vi "Add_Image_Position_Offset.vi"() -> (5 "Plug in titles":string[](array[string]), 7 "Plug in values":string[](array[string]))   [LabVIEW 2020]
uses:
  Utilities/Image acquisition and processing/Feature detection/Typedefs/Theta range.ctl
  Utilities/Image acquisition and processing/Feature detection/Typedefs/Txy range.ctl
  Globals/Meas_global.vi
  Globals/Extra_Commands_Global.vi
  Globals/Trav_pos_global.vi
panel:
  in  "Pre-scale iters":i32=2
  in  "R_min":dbl=200.0
  out "Ty (pixels)":dbl
  out "Tx (pixels)":dbl
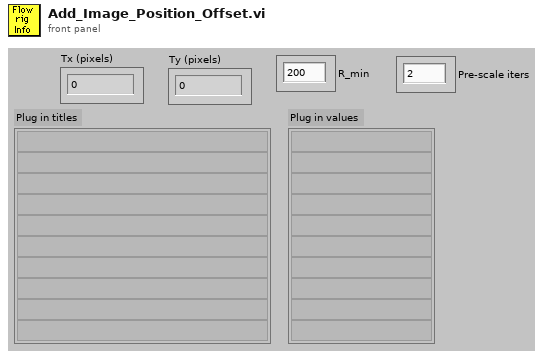
[diagram p1: front panel]
types:
  T1 = typedef "Theta range.ctl" = cluster{"theta max (deg)":dbl, "theta min (deg)":dbl}
  T2 = typedef "Txy range.ctl" = cluster{"Tx max (pix)":i32, "Tx min (pix)":i32, "Ty max (pix)":i32, "Ty min (pix)":i32}
  T3 = cluster{"Tx,y tol (abs pix)":dbl, "Rotation tol (abs deg)":dbl, "Scale tol (rel fact)":dbl}
  T4 = typedef "Post_Process.ctl" = enum16{"Take New Data", "Post Process Raw Data File"}
  T5 = typedef "ROI bounds.ctl" = cluster{"Xmax":i32, "Ymax":i32, "Xmin":i32, "Ymin":i32}
  T6 = typedef "Top level controls.ctl" = cluster{"Auto ROI (for rot.)":bool, "Apply scaling":bool, "Apply rotation":bool, "Apply Tx":bool, "Apply Ty":bool, "Keep proc. img":bool}
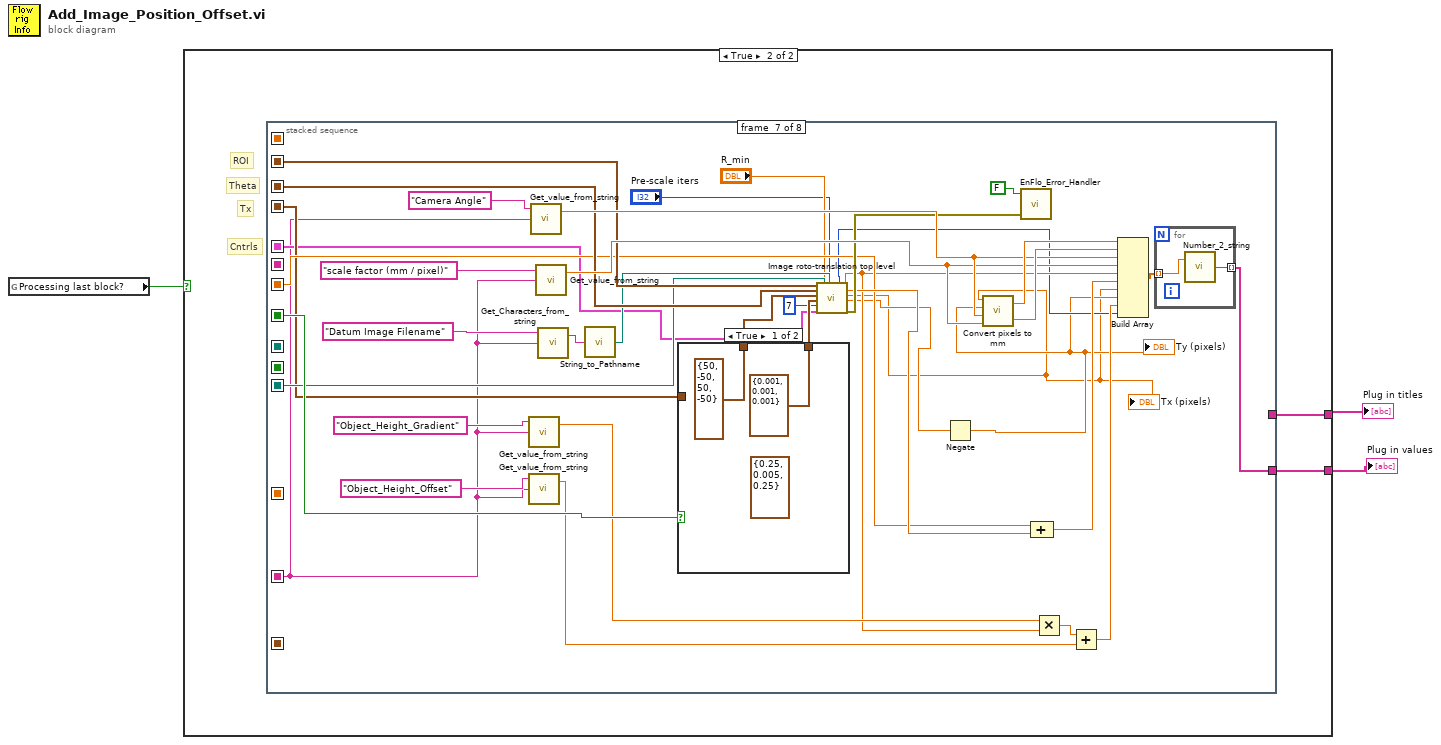
[diagram p0: block diagram]
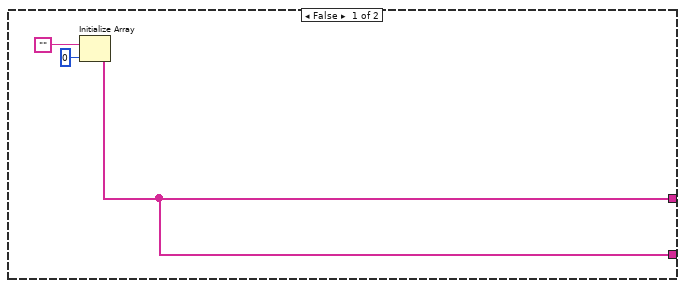
[diagram p2: hidden frame]
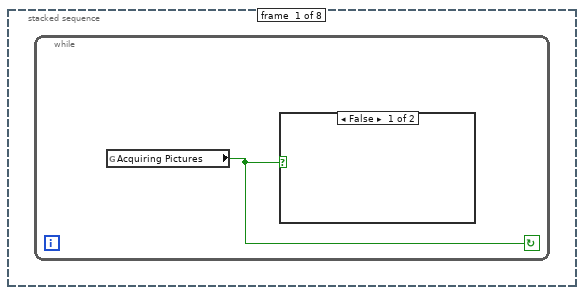
[diagram p3: hidden frame]
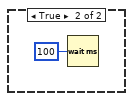
[diagram p4: hidden frame]
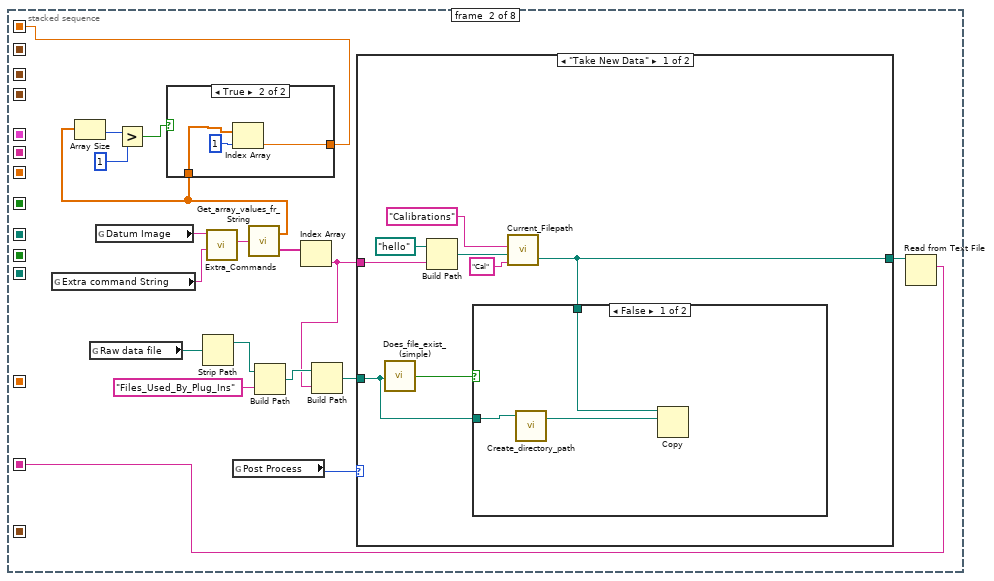
[diagram p5: hidden frame]
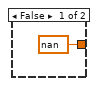
[diagram p6: hidden frame]
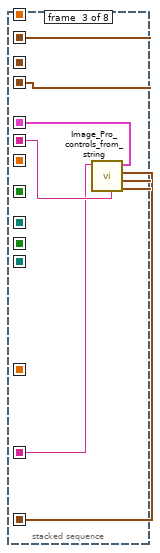
[diagram p9: hidden frame]
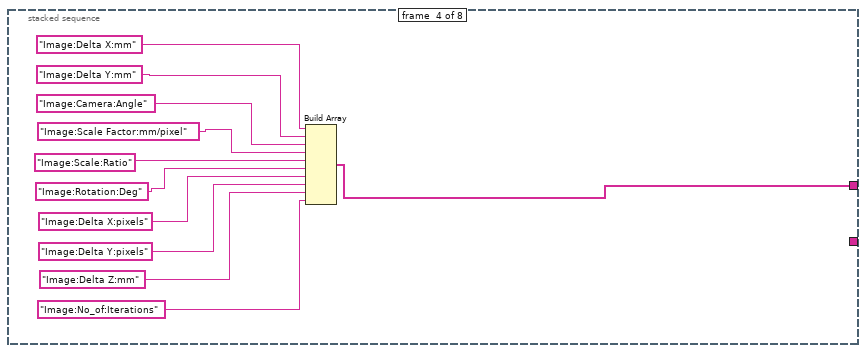
[diagram p10: hidden frame]
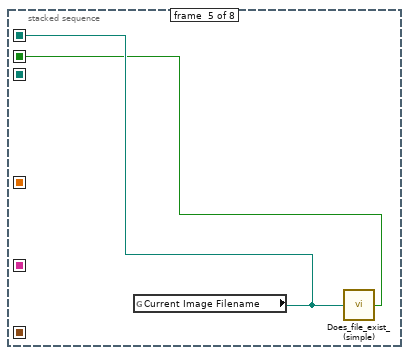
[diagram p11: hidden frame]
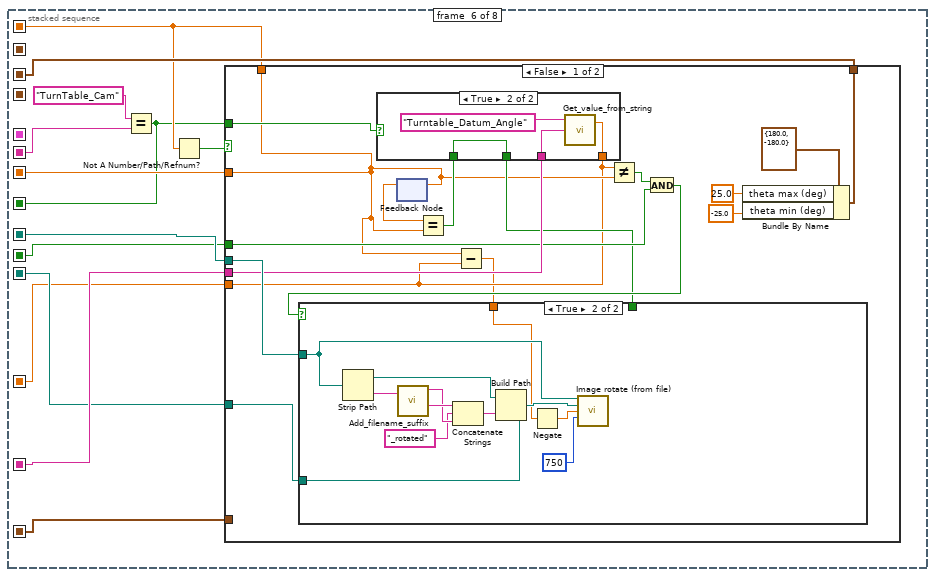
[diagram p12: hidden frame]
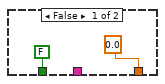
[diagram p13: hidden frame]
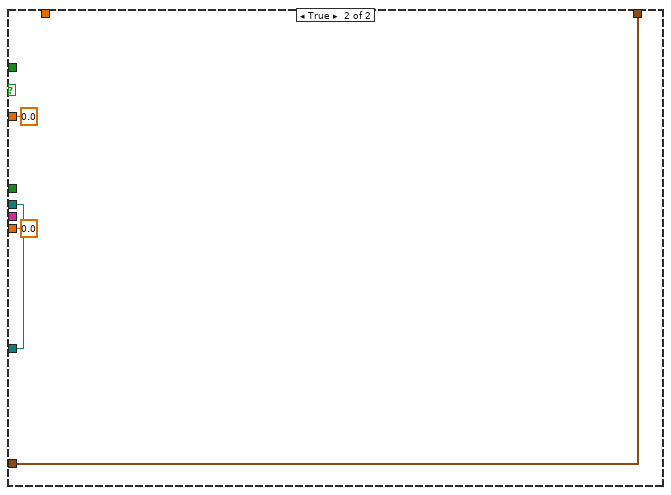
[diagram p15: hidden frame]
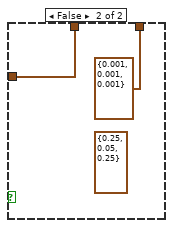
[diagram p16: hidden frame]
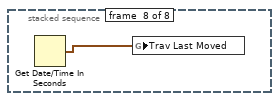
[diagram p17: hidden frame]
diagram:
  n1 = global read "Meas_global.vi" "Processing last block?"() -> (w1:bool)
  n2 = case shown="True" w1 {
    tunnel: [w4 w7] -> w3
    tunnel: [w4 w8] -> w2
    frame False {
      n3 = Initialize Array("", 0) -> (w4:string[])
    }
    frame True {
      # "Theta"
      # "Cntrls"
      # "Tx"
      # "ROI"
      n4 = stacked-sequence {
        seq-local: [_ w26 _ _ _ _ _ _] -> [_ _ w45 _ _ w75 w127 _]
        seq-local: [_ _ w48 _ _ _ _ _] -> [_ _ _ _ _ _ w144 _]
        seq-local: [_ _ _ _ _ w76 _ _] -> [_ _ _ _ _ _ w143 _]
        seq-local: [_ _ _ _ _ w64 _ _] -> [_ _ _ _ _ _ w139 _]
        seq-local: [_ _ _ _ _ w73 _ _] -> [_ _ _ _ _ _ w134 _]
        seq-local: [_ _ _ _ _ w72 _ _] -> [_ _ _ _ _ _ w135 _]
        seq-local: [_ _ w49 _ _ _ _ _] -> [_ _ _ _ _ _ w131 _]
        seq-local: [_ _ w50 _ _ _ _ _] -> [_ _ _ _ _ _ w130 _]
        seq-local: [_ _ _ _ w63 _ _ _] -> [_ _ _ _ _ w71 _ _]
        seq-local: [_ _ _ _ w62 _ _ _] -> [_ _ _ _ _ w70 _ _]
        seq-local: [_ _ _ _ _ w69 _ _] -> [_ _ _ _ _ _ _ _]
        seq-local: [_ _ w47 _ _ _ _ _] -> [_ _ _ _ _ w67 _ _]
        seq-local: [_ _ w46 _ _ _ _ _] -> [_ _ _ _ _ w68 _ _]
        seq-local: [_ w14 _ _ _ _ _ _] -> [_ _ _ _ _ w65 _ _]
        tunnel: [_ _ _ _ _ _ w145 _] -> w8
        tunnel: [_ _ _ w53 _ _ _ _] -> w7
        frame #0 {
          n5 = while {
            stop <- w9 continue-if-true
            n6 = global read "Meas_global.vi" "Acquiring Pictures"() -> (w9:bool)
            n7 = case shown="False" w9 {
              frame False {
              }
              frame True {
                n8 = Wait (ms)(milliseconds to wait=u32 100) -> ()  [unwired: 1 out]
              }
            }
          }
        }
        frame #1 {
          n9 = global read "Meas_global.vi" "Extra command String"() -> (w25:string)
          n10 = global read "Meas_global.vi" "Raw data file"() -> (w22:path)
          n11 = global read "Extra_Commands_Global.vi" "Datum Image"() -> (w28:string)
          n12 = Strip Path(path=w22) -> (stripped path=w21:path)  [unwired: 1 out]
          n13 = call "Extra_Commands.vi"("String to Search"=w25, "Command"=w28) -> ("String Value"=w24:string)  [unwired: 1 in, 4 out]
          n14 = global read "Meas_global.vi" "Post Process"() -> (w16:T4)
          n15 = call "Get_array_values_fr_String.vi"("String Value"=w24) -> ("Numeric Array"=w15:dbl[], "String array"=w23:string[])
          n16 = Array Size(array=w15) -> (size(s)=w13:i32)
          n17 = Greater?(x=w13, y=1) -> (0:w11:bool)
          n18 = case shown="True" w11 {
            tunnel: w15 -> [_ w31]
            tunnel: [nan w30] -> w14
            frame False {
            }
            frame True {
              n19 = Index Array(array=w31, index=1) -> (element=w30:dbl)
            }
          }
          n20 = Build Path(base path=w21, name or relative path="Files_Used_By_Plug_Ins") -> (appended path=w19:path)
          n21 = Index Array(array=w23) -> (element=w18:string)  [unwired: 1 in]
          n22 = Build Path(base path=w19, name or relative path=w18) -> (appended path=w17:path)
          n23 = case shown="\"Take New Data\"" w16 {
            tunnel: [w34 w44] -> w27
            tunnel: w18 -> [w36 _]
            tunnel: w17 -> [w33 w44]
            frame "Take New Data" {
              n24 = call "Does_file_exist_(simple).vi"("Pathname"=w33) -> ("exists?"=w35:bool)
              n25 = Build Path(base path=path "hello", name or relative path=w36) -> (appended path=w40:path)
              n26 = call "Current_Filepath.vi"("Short_Name"="Cal" ("Data Type"), "Filename in"=w40, "Data Type"="Calibrations") -> ("Filename Out"=w34:path)  [unwired: 1 in, 1 out]
              n27 = case shown="False" w35 {
                tunnel: w34 -> [w43 _]
                tunnel: w33 -> [w42 _]
                frame False {
                  n28 = call "Create_directory_path.vi"("Path name"=w42) -> ("Path name Out"=w41:path)  [unwired: 2 in, 1 out]
                  n29 = Copy(10:w41, 11:w43) -> ()  [unwired: 3 in, 3 out]
                }
                frame True {
                }
              }
            }
            frame "Post Process Raw Data File" {
            }
          }
          n30 = Read from Text File(file (use dialog)=w27) -> (text=w26:string)  [unwired: 3 in, 3 out]
        }
        frame #2 {
          n31 = call "Image_Pro_controls_from_string.vi"("Setup String"=w45) -> ("ROI to crop (pixels)"=w48:T5, "Txy range (pixels)"=w49:T2, "Theta range (deg)"=w46:T1, "Controls"=w50:T6, "Camera"=w47:string)  [unwired: 6 in]
        }
        frame #3 {
          n32 = Build Array("Image:Delta X:mm", "Image:Delta Y:mm", "Image:Camera:Angle", "Image:Scale Factor:mm/pixel", "Image:Scale:Ratio", "Image:Rotation:Deg", "Image:Delta X:pixels", "Image:Delta Y:pixels", "Image:Delta Z:mm", "Image:No_of:Iterations") -> (w53:string[])
        }
        frame #4 {
          n33 = global read "Trav_pos_global.vi" "Current Image Filename"() -> (w63:path)
          n34 = call "Does_file_exist_(simple).vi"("Pathname"=w63) -> ("exists?"=w62:bool)
        }
        frame #5 {
          n35 = Equal?(x="TurnTable_Cam", y=w67) -> (x = y?=w64:bool)
          n36 = Not A Number/Path/Refnum?(number/path/refnum=w65) -> (NaN/Path/Refnum?=w66:bool)
          n37 = case shown="False" w66 {
            tunnel: [w92 w112] -> w76
            tunnel: w75 -> [w86 _]
            tunnel: [w89 w115] -> w73
            tunnel: w71 -> [w88 w115]
            tunnel: [w79 sgl 0.0 ("Start X")] -> w72
            tunnel: w70 -> [w84 _]
            tunnel: [w78 0.0 ("Value")] -> w69
            tunnel: w68 -> [_ w112]
            tunnel: w65 -> [w79 _]
            tunnel: w64 -> [w82 _]
            frame False {
              n38 = feedback-in #1(w79) -> ()
              n39 = feedback #1() -> (w87:dbl)  [unwired: 1 in]
              n40 = Equal?(x=w87, y=w79) -> (x = y?=w80:bool)
              n41 = case shown="True" w82 {
                tunnel: w86 -> [_ w98]
                tunnel: [0.0 ("Value") w97] -> w78
                tunnel: [FALSE w96] -> w81
                tunnel: w80 -> [_ w96]
                frame False {
                }
                frame True {
                  n42 = call "Get_value_from_string.vi"("Input string"=w98, "Variable name"="Turntable_Datum_Angle" ("Label for value")) -> ("Value"=w97:dbl)  [unwired: 1 in, 1 out]
                }
              }
              n43 = Subtract(x=w79, y=w78) -> (x-y=w77:dbl)
              n44 = Not Equal?(x=w78, y=w79) -> (x != y?=w85:bool)
              n45 = And(x=w85, y=w84) -> (x .and. y?=w83:bool)
              n46 = case shown="True" w83 {
                tunnel: [w100 w103] -> w89
                tunnel: w88 -> [w100 w105]
                tunnel: w81 -> [_ _]
                tunnel: w77 -> [_ w102]
                frame False {
                }
                frame True {
                  n47 = Strip Path(path=w105) -> (stripped path=w106:path, name=w111:string)
                  n48 = call "Add_filename_suffix.vi"("Filename"=w111) -> ("Original Suffix"=w109:string, "Base name"=w110:string)  [unwired: 1 in, 2 out]
                  n49 = Concatenate Strings(w110, "_rotated" ("string"), w109) -> (w107:string)
                  n50 = Build Path(base path=w106, name or relative path=w107) -> (appended path=w103:path)
                  n51 = Negate(x=w102) -> (-x=w104:dbl)
                  n52 = call "Image rotate (from file).vi"("Image file path"=w105, "Rotated image file path"=w103, "Rotation angle, ccw+ (deg)"=w104, "Quality"=u32 750) -> ()  [unwired: 11 in, 1 out]
                }
              }
              n53 = Bundle By Name(cluster=T1 {"theta max (deg)"=180.0, "theta min (deg)"=-180.0} ("Theta range (deg)"), "theta max (deg)"=25.0, "theta min (deg)"=-25.0) -> (w92:T1)
            }
            frame True {
            }
          }
        }
        frame #6 {
          n54 = call "Get_value_from_string.vi"("Input string"=w127, "Variable name"="Object_Height_Gradient" ("Label for value")) -> ("Value"=w126:dbl)  [unwired: 1 in, 1 out]
          n55 = call "Get_value_from_string.vi"("Input string"=w127, "Variable name"="Object_Height_Offset" ("Label for value")) -> ("Value"=w123:dbl)  [unwired: 1 in, 1 out]
          n56 = call "Get_value_from_string.vi"("Input string"=w127, "Variable name"="Camera Angle" ("Label for value")) -> ("Value"=w148:dbl)  [unwired: 1 in, 1 out]
          n57 = call "Get_value_from_string.vi"("Input string"=w127, "Variable name"="scale factor (mm / pixel)" ("Label for value")) -> ("Value"=w147:dbl)  [unwired: 1 in, 1 out]
          n58 = call "Get_Characters_from_string.vi"("Input string"=w127, "Variable name"="Datum Image Filename" ("Label for characters")) -> ("Value"=w151:string)  [unwired: 1 in, 1 out]
          n59 = call "String_to_Pathname.vi"("Input String"=w151) -> ("path"=w142:path)
          n60 = case shown="True" w139 {
            tunnel: [T3 {"Tx,y tol (abs pix)"=0.001, "Rotation tol (abs deg)"=0.001, "Scale tol (rel fact)"=0.001} ("Convergence tolerances") T3 {"Tx,y tol (abs pix)"=0.001, "Rotation tol (abs deg)"=0.001, "Scale tol (rel fact)"=0.001} ("Convergence tolerances")] -> w136
            tunnel: [T2 {"Tx max (pix)"=50, "Tx min (pix)"=-50, "Ty max (pix)"=50, "Ty min (pix)"=-50} ("Txy range (pixels)") w157] -> w133
            tunnel: w131 -> [_ w157]
            frame True {
              (unwired) T3 {"Tx,y tol (abs pix)"=0.25, "Rotation tol (abs deg)"=0.005, "Scale tol (rel fact)"=0.25} ("Convergence tolerances")
            }
            frame False {
              (unwired) T3 {"Tx,y tol (abs pix)"=0.25, "Rotation tol (abs deg)"=0.05, "Scale tol (rel fact)"=0.25} ("Convergence tolerances")
            }
          }
          n61 = call "Image roto-translation top level.vi"("ROI to crop (pixels)"=w144, "Theta range (deg)"=w143, "Txy range (pixels)"=w133, "Convergence tolerances"=w136, "Max. iters"=7, "Controls"=w130, "Test image file path"=w134, "R_min"="R_min", "Reference image file path"=w142, "Pre-scale iters"="Pre-scale iters") -> ("Iter"=w118:i32, "Scale factor"=w125:dbl, "Rotation (deg)"=w138:dbl, "Tx (pixels)"=w116:dbl, "Ty (pixels)"=w121:dbl, "Error Out"=w141:errorcluster)  [unwired: 2 in, 2 out]
          "Tx (pixels)" <- w116
          n62 = Negate(x=w121) -> (-x=w117:dbl)
          "Ty (pixels)" <- w117
          n63 = call "Convert pixels to mm.vi"("scale factor (mm / pixel)"=w147, "camera angle, ccw+ rel. to trav. (deg)"=w148, "dy (pix)"=w117, "dx (pix)"=w116) -> ("dy (mm)"=w149:dbl, "dx (mm)"=w150:dbl)
          n64 = call "EnFlo_Error_Handler.vi"("error in (no error)"=w141, "Dialog Box (F)"=FALSE ("Dialog Box (T)")) -> ()  [unwired: 2 in, 2 out]
          n65 = Compound Arithmetic op=ADD(w135, w138) -> (w137:dbl)
          n66 = Multiply(x=w126, y=w125) -> (x*y=w124:dbl)
          n67 = Add(x=w124, y=w123) -> (x+y=w122:dbl)
          n68 = Build Array(w150, w149, w148, w147, w125, w137, w116, w117, w122, w118) -> (w146:dbl[])
          n69 = for {
            tunnel: w146 -> [w160] mode=indexing
            tunnel: [w159] -> w145 mode=indexing
            n70 = call "Number_2_string.vi"("number"=w160) -> ("String"=w159:string)  [unwired: 1 in]
          }
        }
        frame #7 {
          n71 = Get Date/Time In Seconds() -> (seconds since 1Jan1904=w161:timestamp)
          n72 = global write "Trav_pos_global.vi" "Trav Last Moved"(w161) -> ()
        }
      }
    }
  }
  "Plug in titles" <- w3
  "Plug in values" <- w2
